vi "CRYSweepCorrCIN.vi"(0 "NOffset":i32, 2 "Deconv Response":cdb[](array[numeric]) format="%.2f", 5 "MStart":dbl, 7 "NHarm":dbl, 9 "MStop":dbl, 11 "Fs":dbl, 12 "FFT size":dbl, 13 "T0":dbl) -> (4 "T0 Position":i32, 6 "FFT Size":i32, 10 "Impulse Response":cdb[](array[numeric]) format="%.2f")   [LabVIEW 2013]
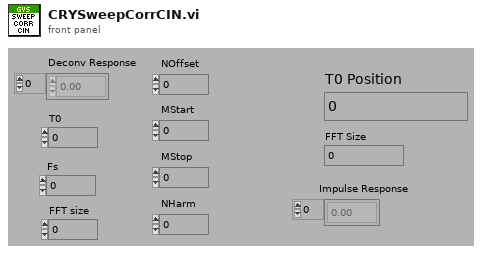
[diagram p1: front panel]
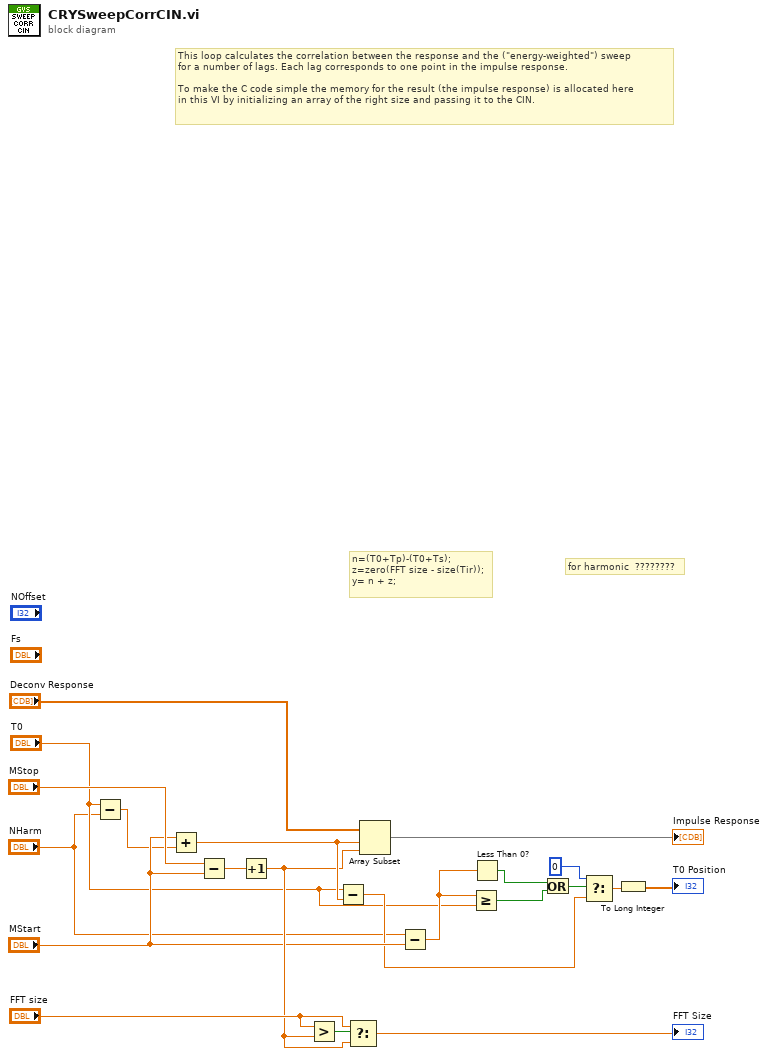
[diagram p0: block diagram]
diagram:
  # "for harmonic  ????????"
  # "n=(T0+Tp)-(T0+Ts);\nz=zero(FFT size - size(Tir));\ny= n + z;"
  # "This loop calculates the correlation between the response and the (\"energy-weighted\") sweep\nfor a number of lags. Each lag corresponds to one point in the impulse response.\n\nTo make the C code simple the memory for the result (the impulse response) is allocated here \nin this VI by initializing an array of the right size and passing it to the CIN."
  n1 = Subtract(x="T0", y="NHarm") -> (x-y=w2:dbl)
  n2 = Add(x="MStart", y=w2) -> (x+y=w19:dbl)
  n3 = Subtract(x="MStop", y="MStart") -> (x-y=w20:dbl)
  n4 = Increment(x=w20) -> (x+1=w16:dbl)
  n5 = Greater?(x="FFT size", y=w16) -> (0:w18:bool)
  n6 = Subtract(x="T0", y=w19) -> (x-y=w9:dbl)
  n7 = Select(t="FFT size", s=w18, f=w16) -> (s? t:f=→"FFT Size":dbl)
  n8 = Array Subset(array="Deconv Response", index=w19, length=w16) -> (→"Impulse Response":cdb[])
  n9 = Subtract(x="NHarm", y="MStart") -> (x-y=w13:dbl)
  n10 = Greater Or Equal?(x=w13, y="T0") -> (x >= y?=w10:bool)
  n11 = Less Than 0?(x=w13) -> (x < 0?=w11:bool)
  n12 = Or(x=w11, y=w10) -> (x .or. y?=w12:bool)
  n13 = Select(t=0 ("T0 Position"), s=w12, f=w9) -> (s? t:f=w7:dbl)
  n14 = To Long Integer(number=w7) -> (32bit integer=→"T0 Position":i32)
